vi "Receive And Get Parameter.vi"(8 "error in (no error)":errorcluster, 10 "timeout in ms (-1)":i32=-1, 11 "result_from_call in":refnum<class "result_from_call.lvclass">) -> (0 "error out":errorcluster, 1 "timeout":bool, 2 "Data":variant, 3 "result_from_call out":refnum<class "result_from_call.lvclass">)   [LabVIEW 2015, in "result_from_call.lvclass"]
uses:
  result_from_call.lvclass
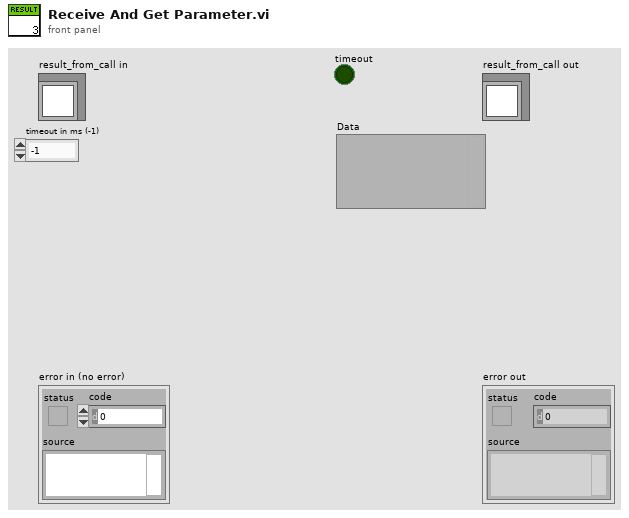
[diagram p1: front panel]
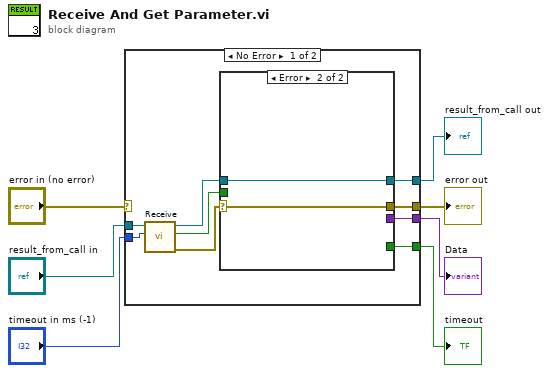
[diagram p0: block diagram]
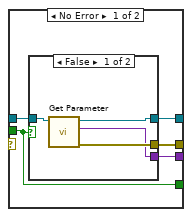
[diagram p2: hidden frame]
diagram:
  n1 = case shown="No Error" "error in (no error)" {
    selector: "error in (no error)" -> [_ w30]
    tunnel: [w13 w30] -> w6
    tunnel: [w12 w29] -> w4
    tunnel: "result_from_call in" -> [w16 w29]
    tunnel: [w10 _] -> w1
    tunnel: [w9 _] -> w2
    tunnel: "timeout in ms (-1)" -> [w8 _]
    frame No Error {
      n2 = call "Receive.vi"("timeout in ms (-1)"=w8, "result_from_call in"=w16) -> ("error out"=w11:errorcluster, "timeout"=w15:bool, "result_from_call out"=w14:refnum<class "result_from_call.lvclass">)  [unwired: 7 in]
      n3 = case shown="Error" w11 {
        selector: w11 -> [_ w27]
        tunnel: w15 -> [w17 _]
        tunnel: w14 -> [w21 w28]
        tunnel: [w20 w27] -> w13
        tunnel: [w19 w28] -> w12
        tunnel: [w18 _] -> w10
        tunnel: [w17 _] -> w9
        frame No Error {
          n4 = case shown="False" w17 {
            tunnel: w21 -> [w25 w26]
            tunnel: [w24 _] -> w20
            tunnel: [w23 w26] -> w19
            tunnel: [w22 _] -> w18
            frame False {
              n5 = call-dynamic "Get Parameter.vi"("result_from_call in"=w25) -> ("error out"=w24:errorcluster, "Data"=w22:variant, "result_from_call out"=w23:refnum<class "result_from_call.lvclass">)  [unwired: 8 in]
            }
            frame True {
            }
          }
        }
        frame Error {
        }
      }
    }
    frame Error {
    }
  }
  "error out" <- w6
  "result_from_call out" <- w4
  "timeout" <- w2
  "Data" <- w1
